vi "Measurement Logic.vi"() -> ()   [LabVIEW 2020, in "UIProgressUpdates.lvlib"]
uses:
  UIProgressUpdates.lvlib
  Measurement Configuration.ctl
  Measurement Results.ctl
  <vilib>/MeasurementLink/MeasurementLink Measurement Server/Classes/MeasurementContext/MeasurementContext.lvclass
  <vilib>/MeasurementLink/MeasurementLink Measurement Server/Classes/MeasurementContext/Accessor/Is Canceled.vi
panel:
  out "Measurement Context out":refnum<class "MeasurementContext.lvclass">
  in  "Measurement Context":refnum<class "MeasurementContext.lvclass">
  out "Measurement Results":T1
  in  "Measurement Configuration":T2
  out "error out":errorcluster
  in  "error in":errorcluster
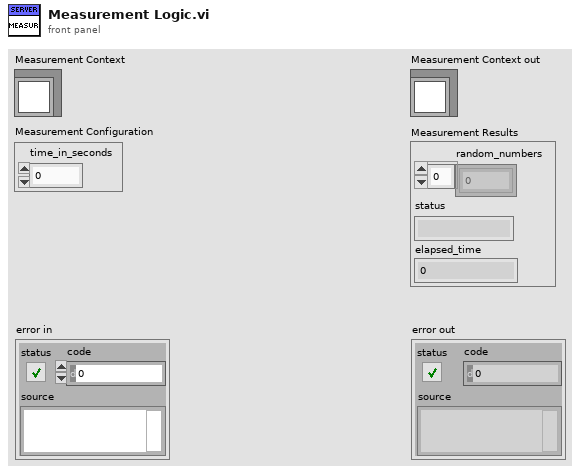
[diagram p1: front panel]
types:
  T1 = typedef "UIProgressUpdates.lvlib/Measurement Results.ctl" = cluster{"random_numbers":dbl[], "status":string, "elapsed_time":dbl}
  T2 = typedef "UIProgressUpdates.lvlib/Measurement Configuration.ctl" = cluster{"time_in_seconds":dbl}
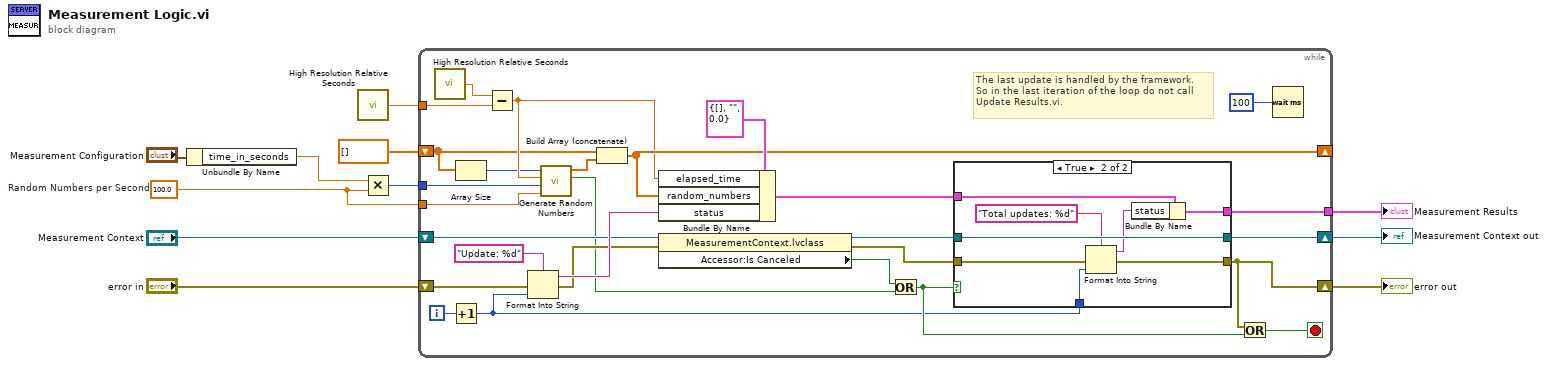
[diagram p0: block diagram]
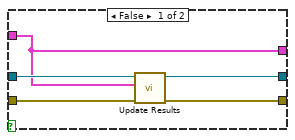
[diagram p2: hidden frame]
diagram:
  w2 = 100.0  # Random Numbers per Second
  n1 = Unbundle By Name("Measurement Configuration") -> ("time_in_seconds"=w3:dbl)
  n2 = call <vilib>:"High Resolution Relative Seconds.vi"() -> ("relative seconds"=w4:dbl)
  n3 = Multiply(x=w3, y=w2) -> (x*y=w1:i32)
  n4 = while {
    shift-right: [w30] -> w9
    shift-left: "Measurement Context" -> [w35]
    shift-right: [w29] -> w8
    shift-left: "error in" -> [w38]
    shift-right: [w18] -> _
    shift-left: dbl[] [] -> [w16]
    tunnel: [w25] -> w5
    tunnel: w4 -> [w21]
    tunnel: w2 -> [w12]
    tunnel: w1 -> [w13]
    i -> [w24]
    stop <- w26 stop-if-true
    # "The last update is handled by the framework.\nSo in the last iteration of the loop do not call\nUpdate Results.vi."
    n5 = call <vilib>:"High Resolution Relative Seconds.vi"() -> ("relative seconds"=w22:dbl)
    n6 = Increment(x=w24) -> (x+1=w20:i32)
    n7 = Array Size(array=w16) -> (size(s)=w15:i32)
    n8 = Subtract(x=w22, y=w21) -> (x-y=w17:dbl)
    n9 = Format Into String(format string="Update: %d", error in=w38, w20) -> (resulting string=w37:string, error out=w34:errorcluster)  [unwired: 1 in]
    n10 = call "Generate Random Numbers.vi"("Random Numbers per Second"=w12, "Stop Length"=w13, "Elapsed Time"=w17, "Current Array Size"=w15) -> ("Done?"=w14:bool, "Random Numbers out"=w27:dbl[])  [unwired: 6 in]
    n11 = Build Array (concatenate)(w16, w27) -> (w18:dbl[])
    n12 = Bundle By Name(cluster=T1 {"random_numbers"=[], "status"="", "elapsed_time"=0.0} ("Measurement Results"), "elapsed_time"=w17, "random_numbers"=w18, "status"=w37) -> (w28:T1)
    n13 = property class="MeasurementContext.lvclass"(reference=w35, error in=w34) -> (reference out=w33:refnum<class "MeasurementContext.lvclass">, error out=w32:errorcluster, "Accessor:Is Canceled"=w31:bool)
    n14 = Or(x=w31, y=w14) -> (x .or. y?=w23:bool)
    n15 = case shown="True" w23 {
      tunnel: w33 -> [w44 w52]
      tunnel: w32 -> [w43 w49]
      tunnel: [w41 w52] -> w30
      tunnel: [w42 w48] -> w29
      tunnel: w28 -> [w40 w51]
      tunnel: [w40 w50] -> w25
      tunnel: w20 -> [_ w45]
      frame False {
        n16 = call <vilib>:"Update Results.vi"("error in (no error)"=w43, "Measurement Results"=w40, "MeasurementContext in"=w44) -> ("error out"=w42:errorcluster, "MeasurementContext out"=w41:refnum<class "MeasurementContext.lvclass">)  [unwired: 7 in]
      }
      frame True {
        n17 = Format Into String(format string="Total updates: %d" ("status"), error in=w49, w45) -> (resulting string=w46:string, error out=w48:errorcluster)  [unwired: 1 in]
        n18 = Bundle By Name(cluster=w51, "status"=w46) -> (w50:T1)
      }
    }
    n19 = Or(x=w29, y=w23) -> (x .or. y?=w26:bool)
    n20 = Wait (ms)(milliseconds to wait=u32 100 ("UI Update Interval (msec)")) -> ()  [unwired: 1 out]
  }
  "error out" <- w8
  "Measurement Results" <- w5
  "Measurement Context out" <- w9
